vi "Map XY To Coords.vi"(7 "Y Scale":i32, 8 "error in (no error)":errorcluster, 9 "X Scale":i32, 10 "XY":cluster{"X":dbl, "Y":dbl}, 11 "GraphChart in":refnum<class "GraphChart.lvclass">) -> (0 "error out":errorcluster, 1 "Coords":T1, 2 "Map XY To Coordinates":bool, 3 "GraphChart out":refnum<class "GraphChart.lvclass">)   [LabVIEW 2015, in "GraphChart.lvclass"]
doc: "Returns TRUE and maps the XY location on a graph to the owning pane coordinates. If you do not specify the scales, LabVIEW uses the active or current scales. This method is useful when you need to map graph coordinates to plot image coordinates to draw images inside the plot area of a graph.\n\n This method adjusts only the left and top plot bounds to orient the plot around the origin of the owning pane.\n\nQControl Class wrapper around the <b>GraphChart : Map XY To Coordinates Method</b>.\n<b> </b> <b> </b>\n©2016 Q Software Innovations, LLC (QSI)\nwritten by Quentin Alldredge\nproduced in LabVIEW 2015\n\nsupport@qsoftwareinnovations.com\nwww.qsoftwareinnovations.com\n\nAll rights reserved.\n\nRedistribution and use in source and binary forms, with or without modification, are permitted provided that the following conditions are met:\n\n * Redistributions of source code must retain the above copyright notice, this list of conditions and the following disclaimer.\n * Redistributions in binary form must reproduce the above copyright notice, this list of conditions and the following disclaimer in the documentation and/or other materials provided with the distribution.\n * Neither the name of Q Software Innovations, LLC. nor the names of its contributors may be used to endorse or promote products derived from this software without specific prior written permission.\n\nTHIS SOFTWARE IS PROVIDED BY THE COPYRIGHT HOLDERS AND CONTRIBUTORS \"AS IS\" AND ANY EXPRESS OR IMPLIED WARRANTIES, INCLUDING, BUT NOT LIMITED TO, THE IMPLIED WARRANTIES OF MERCHANTABILITY AND FITNESS FOR A PARTICULAR PURPOSE ARE DISCLAIMED. IN NO EVENT SHALL THE COPYRIGHT OWNER OR CONTRIBUTORS BE LIABLE FOR ANY DIRECT, INDIRECT, INCIDENTAL, SPECIAL, EXEMPLARY, OR CONSEQUENTIAL DAMAGES (INCLUDING, BUT NOT LIMITED TO, PROCUREMENT OF SUBSTITUTE GOODS OR SERVICES; LOSS OF USE, DATA, OR PROFITS; OR BUSINESS INTERRUPTION) HOWEVER CAUSED AND ON ANY THEORY OF LIABILITY, WHETHER IN CONTRACT, STRICT LIABILITY, OR TORT (INCLUDING NEGLIGENCE OR OTHERWISE) ARISING IN ANY WAY OUT OF THE USE OF THIS SOFTWARE, EVEN IF ADVISED OF THE POSSIBILITY OF SUCH DAMAGE."
uses:
  GraphChart.lvclass
  <vilib>/Utility/miscctls.llb/LVPoint32TypeDef.ctl
  GraphChart.lvclass/GraphChart.ctl
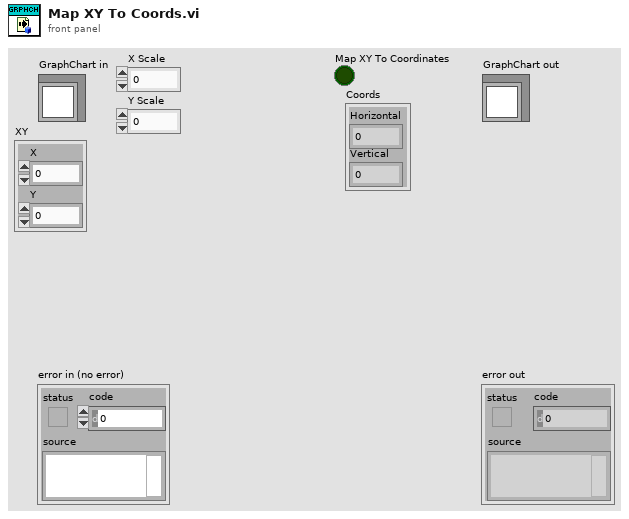
[diagram p1: front panel]
types:
  T1 = typedef "LVPoint32TypeDef.ctl" = cluster{"Horizontal":i32, "Vertical":i32}
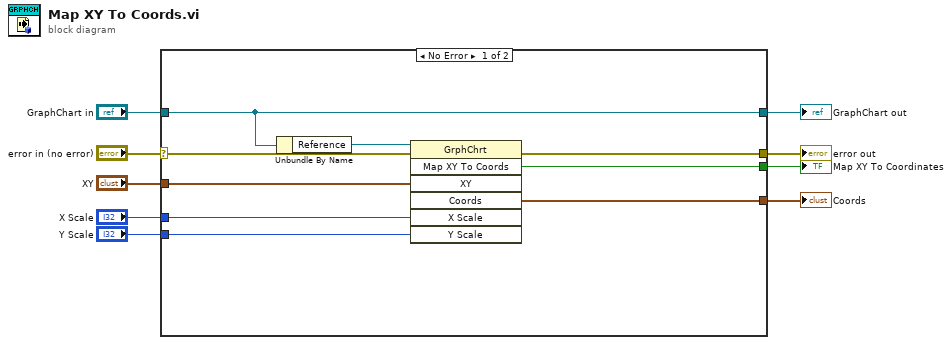
[diagram p0: block diagram]
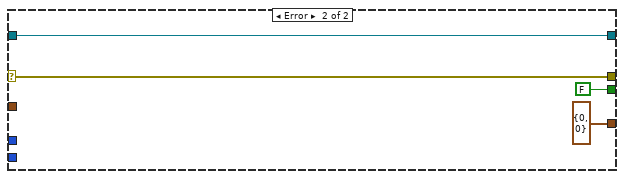
[diagram p2: hidden frame]
diagram:
  n1 = case shown="No Error" "error in (no error)" {
    selector: "error in (no error)" -> [w18 w22]
    tunnel: [w17 w22] -> w8
    tunnel: [w16 w21] -> w6
    tunnel: "GraphChart in" -> [w16 w21]
    tunnel: "XY" -> [w14 _]
    tunnel: [w13 FALSE ("Map XY To Coords")] -> w4
    tunnel: "X Scale" -> [w12 _]
    tunnel: [w11 T1 {"Horizontal"=0, "Vertical"=0} ("Coords")] -> w2
    tunnel: "Y Scale" -> [w10 _]
    frame No Error {
      n2 = Unbundle By Name(w16) -> ("Reference"=w15:refnum<vi>)
      n3 = invoke class="GrphChrt" method="Map XY To Coords"(reference=w15, error in=w18, "XY"=w14, "X Scale"=w12, "Y Scale"=w10) -> (error out=w17:errorcluster, "Map XY To Coords"=w13:bool, "Coords"=w11:T1)  [unwired: 2 in, 4 out]
    }
    frame Error {
    }
  }
  "error out" <- w8
  "GraphChart out" <- w6
  "Map XY To Coordinates" <- w4
  "Coords" <- w2
